vi "outgoing data.vi"(6 "timeout (-1)":i32=-1, 8 "error in":errorcluster, 11 "websocket user plugin in":refnum<class "websocket user plugin.lvclass">) -> (0 "error out":errorcluster, 1 "timeout":bool, 2 "opcode":u8=1, 3 "data":string, 5 "not last fragment (F)":bool)   [LabVIEW 2013, in "websocket user plugin.lvclass"]
uses:
  websocket user plugin.lvclass
  opcode.ctl
  websocket upgrade handler.lvclass
panel:
  in  "send":bool
  in  "opcode 2":T1=1 items=["text"=1, "binary"=2, "x3"=3, "x4"=4, "x5"=5, "x6"=6, "x7"=7]
  in  "data 2":string
  in  "not last fragment (F) 2":bool
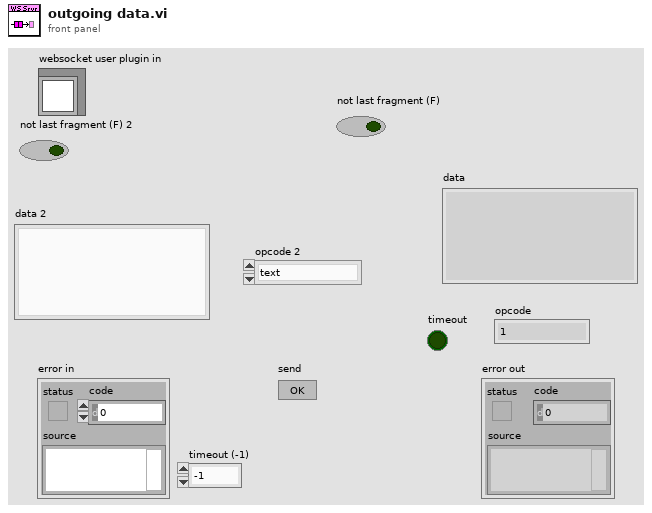
[diagram p1: front panel]
types:
  T1 = typedef "websocket upgrade handler.lvclass/opcode.ctl" = u8
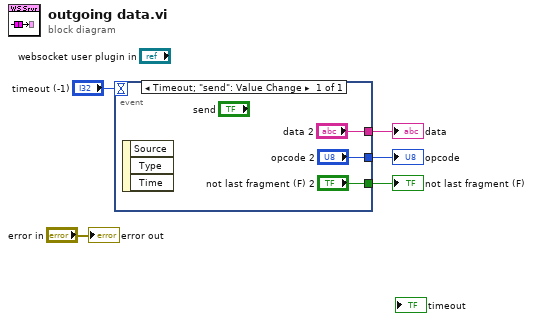
[diagram p0: block diagram]
diagram:
  n1 = event shown="[0] Timeout;  \"send\": Value Change" {
    selector: _ -> [_]
    dyn-events: _ -> [_]
    timeout: "timeout (-1)" -> [_]
    tunnel: ["data 2"] -> w3
    tunnel: ["opcode 2"] -> w2
    tunnel: ["not last fragment (F) 2"] -> w1
    event Timeout; "send": Value Change {
      n2 = event-data() -> ()  [unwired: 1 in, 3 out]
    }
  }
  "data" <- w3
  "opcode" <- w2
  "not last fragment (F)" <- w1
  "error out" <- "error in"
